vi "create.include_task.vi"(10 "topic":string[](array[string])) -> (3 "Include Filter":refnum<class "include.lvclass">)   [LabVIEW 2020, in "nominal types.lvlib" / "channelFilter.lvlib" / "channelFilter.lvclass"]
uses:
  channelFilter.lvclass
  include/include.lvclass
  topic/topic.lvclass
  C:/code/labview-client/lv_src/nominal types/filterTypes/filterTypes.lvclass
  topic/topic.lvclass/topic.ctl
  include/include.lvclass/include.ctl
  topic/topic.set.vi
  include/include.set.vi
  filterTypes/filterTypes.lvclass
  channelFilter.lvclass/channelFilter.ctl
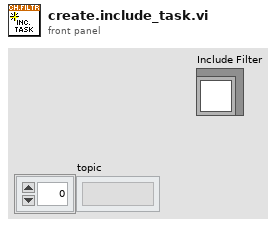
[diagram p1: front panel]
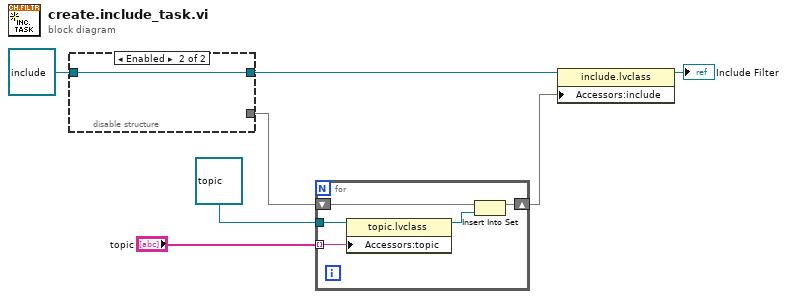
[diagram p0: block diagram]
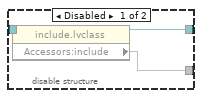
[diagram p2: hidden frame]
diagram:
  n1 = disable-structure shown="Enabled" {
    disable-tunnel: refnum<class "include.lvclass"> refnum ("nominal types.lvlib:channelFilter.lvlib:include.lvclass") -> [w10 w11]
    disable-tunnel: [w9 w11] -> w2
    disable-tunnel: [w8 _] -> w1
    frame Disabled {
      n2 = property class="include.lvclass"(reference=w10) -> (reference out=w9:refnum<class "include.lvclass">, "Accessors:include"=w8:set{refnum<class "filterTypes.lvclass">})  [unwired: 1 in, 1 out]
    }
    frame Enabled {
    }
  }
  n3 = for {
    tunnel: refnum<class "topic.lvclass"> refnum ("nominal types.lvlib:channelFilter.lvlib:topic.lvclass") -> [w16]
    shift-right: [w13] -> w7
    shift-left: w1 -> [w15]
    tunnel: "topic" -> [w12] mode=indexing
    n4 = property class="topic.lvclass"(reference=w16, "Accessors:topic"=w12) -> (reference out=w14:refnum<class "topic.lvclass">)  [unwired: 1 in, 1 out]
    n5 = Insert Into Set(10:w14, 11:w15) -> (3:w13:set{refnum<class "filterTypes.lvclass">})  [unwired: 1 out]
  }
  n6 = property class="include.lvclass"(reference=w2, "Accessors:include"=w7) -> (reference out=→"Include Filter":refnum<class "include.lvclass">)  [unwired: 1 in, 1 out]
